vi "Setpoint.vi"   [LabVIEW 2012, in "Roboteq.lvlib"]
uses:
  Roboteq.lvlib
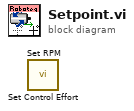
[diagram p0: block diagram]
diagram:
  n1 = call "Set Control Effort.vi"() -> ()  [unwired: 9 in, 3 out]
  n2 = call "Set RPM.vi"() -> ()  [unwired: 9 in, 3 out]
